vi "MultiLayerPerceptron.vi"   [LabVIEW 2020]
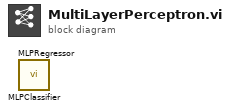
[diagram p0: block diagram]
diagram:
  n1 = call "MLPClassifier.vi"() -> ()  [unwired: 10 in, 2 out]
  n2 = call "MLPRegressor.vi"() -> ()  [unwired: 10 in, 2 out]
